vi "input.vi"(8 "error in":errorcluster, 10 "data table in":T1, 11 "Modbus Slave runtime in":refnum<class "Modbus Slave runtime.lvclass">) -> (0 "error out":errorcluster, 2 "data table out":T1, 3 "Modbus Slave runtime out":refnum<class "Modbus Slave runtime.lvclass">)   [LabVIEW 2013, in "Modbus Slave runtime.lvclass"]
doc: "Provides an interface for reading data from a module at runtime. While this interface performs no operations, a child should provide an override which may read from any open sessions, references, or interfaces.Platypus Framework 1.0.1.65\nNI Systems Engineering - National Instruments"
uses:
  Modbus Slave runtime.lvclass
  <vilib>/NI/Tag Bus/table/data table.ctl
  Modbus Slave runtime.lvclass/Modbus Slave runtime.ctl
  <vilib>/NI/Modbus Library/API/Modbus API.lvclass
  <vilib>/NI/Tag Bus/table/data table.lvlib
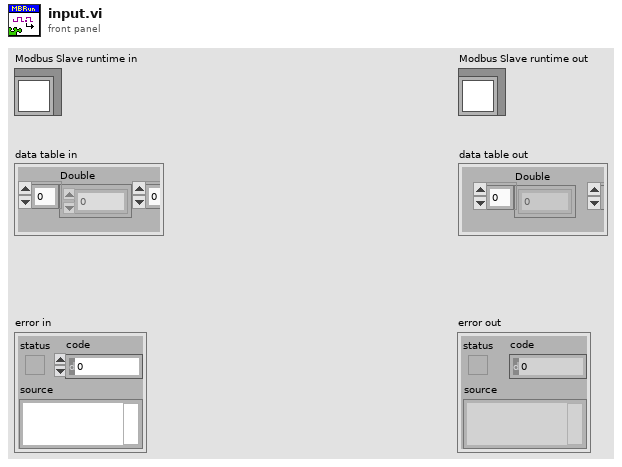
[diagram p1: front panel]
types:
  T1 = typedef "tag bus.lvlib/data table.lvlib/data table.ctl" = cluster{"Double":dbl[], "Single":sgl[], "I64":i64[], "I32":i32[], "I16":i16[], "I8":i8[], "U64":u64[], "U32":u32[], "U16":u16[], "U8":u8[], "Boolean":bool[], "String":string[], "Array of Double":cluster{"DBL Array":dbl[]}[], "Array of Single":cluster{"SGL Array":sgl[]}[], "Array of I64":cluster{"I64 Array":i64[]}[], "Array of I32":cluster{"I32 Array":i32[]}[], "Array of I16":cluster{"I16 Array":i16[]}[], "Array of I8":cluster{"I8 Array":i8[]}[], "Array of U64":cluster{"U64 Array":u64[]}[], "Array of U32":cluster{"U32 Array":u32[]}[], "Array of U16":cluster{"U16 Array":u16[]}[], "Array of U8":cluster{"U8 Array":u8[]}[], "Array of Boolean":cluster{"Boolean Array":bool[]}[], "Array of String":cluster{"String Array":string[]}[]}
  T2 = typedef "Modbus Slave runtime.lvclass/bulk data access.ctl" = cluster{"modbus type":T3, "start":u16, "length":u16, "maps":T4[]}
  T3 = typedef "Modbus Module Channel.lvclass/data bank type.ctl" = enum16{"coils", "discrete inputs", "input registers", "holding registers"}
  T4 = typedef "Modbus Slave runtime.lvclass/data mapping elements.ctl" = cluster{"data type":T5, "data index":i32, "element index":i32, "subindex":i32}
  T5 = typedef "tag bus.lvlib/tag descriptor.lvclass/Data Type.ctl" = enum16{"Double", "Single", "I64", "I32", "I16", "I8", "U64", "U32", "U16", "U8", "Boolean", "String", "Array of Double", "Array of Single", "Array of I64", "Array of I32", "Array of I16", "Array of I8", "Array of U64", "Array of U32", "Array of U16", "Array of U8", "Array of Boolean", "Array of String"}
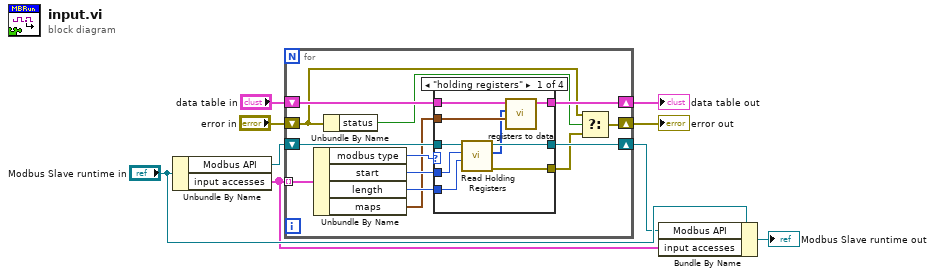
[diagram p0: block diagram]
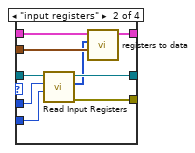
[diagram p2: hidden frame]
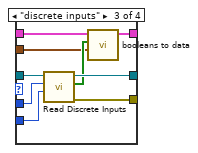
[diagram p3: hidden frame]
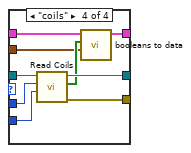
[diagram p4: hidden frame]
diagram:
  n1 = Unbundle By Name("Modbus Slave runtime in") -> ("Modbus API"=w7:refnum<class "Modbus API.lvclass">, "input accesses"=w1:T2[])
  n2 = for {
    shift-right: [w20] -> w6
    shift-left: w7 -> [w21]
    shift-right: [w22] -> w4
    shift-left: "error in" -> [w11]
    tunnel: w1 -> [w18] mode=indexing
    shift-right: [w13] -> w2
    shift-left: "data table in" -> [w14]
    n3 = Unbundle By Name(w18) -> ("modbus type"=w15:T3, "start"=w16:u16, "length"=w17:u16, "maps"=w12:T4[])
    n4 = Unbundle By Name(w11) -> ("status"=w10:bool)
    n5 = case shown="\"holding registers\"" w15 {
      tunnel: w21 -> [w29 w38 w47 w56]
      tunnel: [w31 w40 w49 w58] -> w20
      tunnel: [w30 w39 w48 w57] -> w19
      tunnel: w16 -> [w28 w37 w46 w55]
      tunnel: w17 -> [w27 w36 w45 w54]
      tunnel: w14 -> [w26 w35 w44 w52]
      tunnel: [w25 w34 w43 w53] -> w13
      tunnel: w12 -> [w24 w33 w41 w50]
      frame "holding registers" {
        n6 = call-dynamic "Read Holding Registers.vi"("number of inputs"=w27, "starting address"=w28, "Modbus instance in"=w29) -> ("error out"=w30:errorcluster, "register values"=w23:u16[], "Modbus instance out"=w31:refnum<class "Modbus API.lvclass">)  [unwired: 6 in]
        n7 = call "registers to data.vi"("specifications"=w24, "registers"=w23, "allocation"=w26) -> ("data table"=w25:T1)  [unwired: 8 in]
      }
      frame "input registers" {
        n8 = call-dynamic "Read Input Registers.vi"("number of inputs"=w36, "starting address"=w37, "Modbus instance in"=w38) -> ("error out"=w39:errorcluster, "register values"=w32:u16[], "Modbus instance out"=w40:refnum<class "Modbus API.lvclass">)  [unwired: 6 in]
        n9 = call "registers to data.vi"("specifications"=w33, "registers"=w32, "allocation"=w35) -> ("data table"=w34:T1)  [unwired: 8 in]
      }
      frame "discrete inputs" {
        n10 = call-dynamic "Read Discrete Inputs.vi"("number of inputs"=w45, "starting address"=w46, "Modbus instance in"=w47) -> ("error out"=w48:errorcluster, "discrete inputs"=w42:bool[], "Modbus instance out"=w49:refnum<class "Modbus API.lvclass">)  [unwired: 6 in]
        n11 = call "booleans to data.vi"("specifications"=w41, "booleans"=w42, "allocation"=w44) -> ("data table"=w43:T1)  [unwired: 8 in]
      }
      frame "coils" {
        n12 = call-dynamic "Read Coils.vi"("number of inputs"=w54, "starting address"=w55, "Modbus instance in"=w56) -> ("error out"=w57:errorcluster, "coils"=w51:bool[], "Modbus instance out"=w58:refnum<class "Modbus API.lvclass">)  [unwired: 6 in]
        n13 = call "booleans to data.vi"("specifications"=w50, "booleans"=w51, "allocation"=w52) -> ("data table"=w53:T1)  [unwired: 8 in]
      }
    }
    n14 = Select(t=w11, s=w10, f=w19) -> (s? t:f=w22:errorcluster)
  }
  "error out" <- w4
  "data table out" <- w2
  n15 = Bundle By Name(cluster="Modbus Slave runtime in", "Modbus API"=w6, "input accesses"=w1) -> (→"Modbus Slave runtime out":refnum<class "Modbus Slave runtime.lvclass">)
